vi "Get Interface Settings - Controls Detail Level.vi"(8 "error in (no error)":errorcluster {"code" format="Error %.0f"}, 11 "VIDoc Printer In":refnum<class "VIDoc Printer.lvclass">) -> (0 "error out":errorcluster {"code" format="Error %.0f"}, 2 "Detail Level":T1, 3 "VIDoc Printer Out":refnum<class "VIDoc Printer.lvclass">)   [LabVIEW 2023, in "VIDoc Printer.lvlib" / "VIDoc Printer.lvclass"]
uses:
  VIDoc Printer.lvclass
  Settings/Printer Settings/Detail Level Enum.ctl
  VIDoc Printer.lvclass/VIDoc Printer.ctl
  Settings/Printer Settings/Printer Settings.lvclass
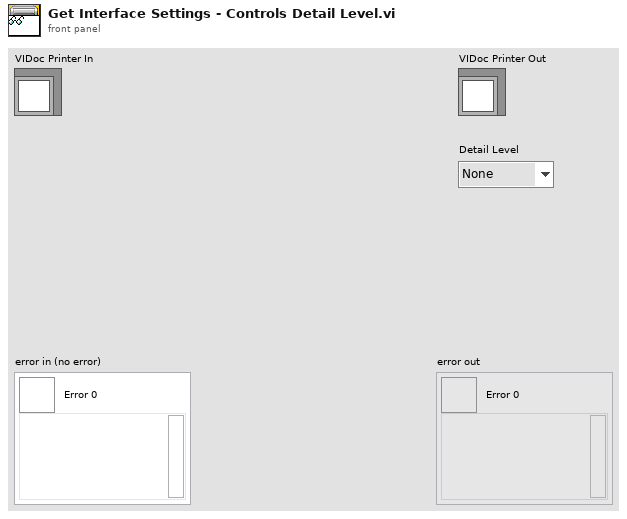
[diagram p1: front panel]
types:
  T1 = typedef "VIDoc Printer.lvlib/Printer Settings.lvclass/Detail Level Enum.ctl" = enum16{"None", "Minimal", "Standard", "Full"}
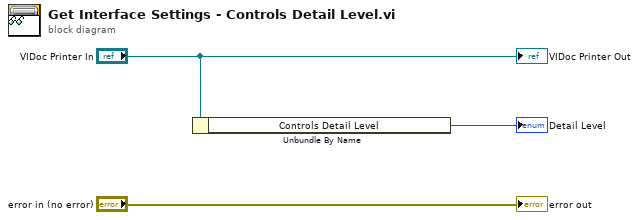
[diagram p0: block diagram]
diagram:
  n1 = Unbundle By Name("VIDoc Printer In") -> ("Controls Detail Level"=→"Detail Level":T1)
  "error out" <- "error in (no error)"
  "VIDoc Printer Out" <- "VIDoc Printer In"
